vi "DPSK_RECV_TEST.vi"() -> ()   [LabVIEW 2020]
uses:
  <vilib>/Utility/error.llb/DialogType.ctl
  <instrlib>/niUSRP/niUSRP Fetch Rx Data (CDB WDT).vi
panel:
  in  "数据源文件":path=path "C:/Users/admin/Desktop/USRP0902/USRP/Dpsk/SendBit.mat"
  in  "接收码元速率":dbl=10000.0
  in  "信源比特长度":dbl=1000.0
  out "波形图":dbl[](graph)
  in  "Stop Button":bool
  in  "天线选择":string="RX2"
  out "实际接收增益":dbl=10.0 format="%#_6f"
  out "实际载波频率":dbl=1000000000.0 format="%#_6p"
  out "实际基带采样率":dbl=200000.0 format="%#_6p"
  in  "设定接收增益":dbl=10.0 format="%#_6f"
  in  "设定载波频率":dbl=1000000000.0 format="%#_6p"
  in  "设定基带采样率":dbl=200000.0 format="%#_6p"
  in  "设备IP":refnum<k15>="192.168.10.2"
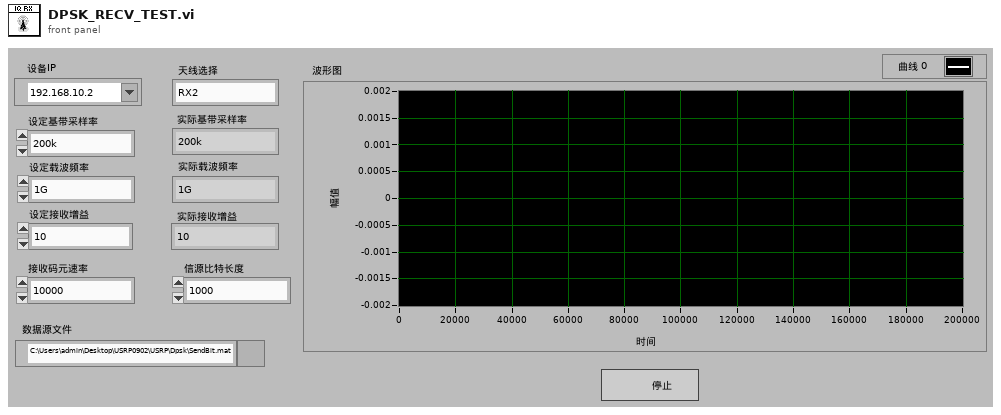
[diagram p1: front panel]
types:
  T1 = typedef "DialogType.ctl" = u16
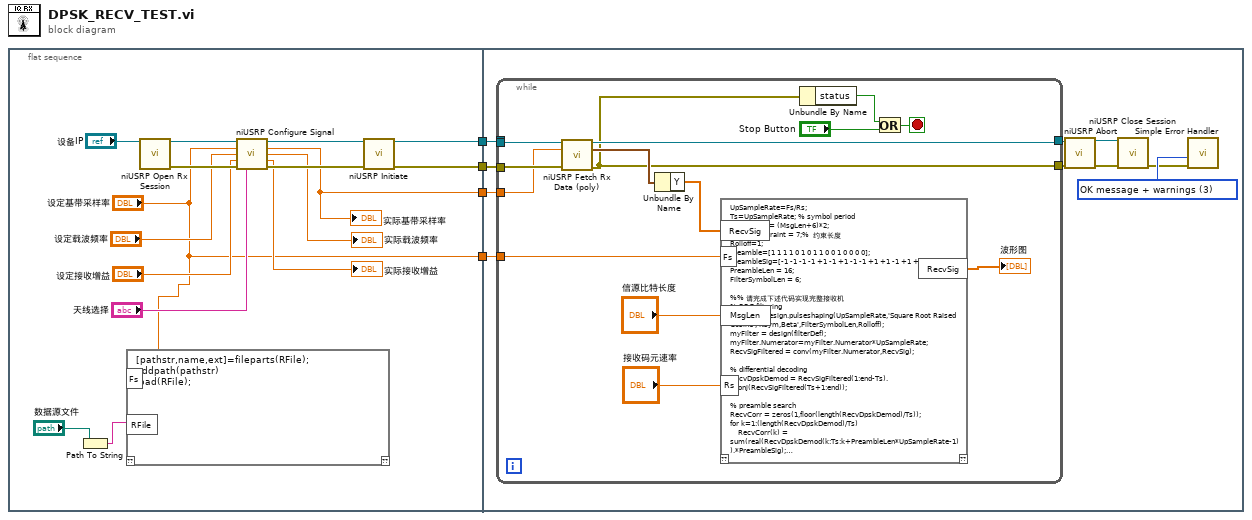
[diagram p0: block diagram]
diagram:
  n1 = flat-sequence {
    tunnel: [w11] -> w4
    tunnel: [w10] -> w3
    tunnel: ["设定基带采样率"] -> w2
    tunnel: [w9] -> w1
    tunnel: w4 -> [w26]
    tunnel: w3 -> [w25]
    tunnel: w2 -> [w22]
    tunnel: w1 -> [w21]
    frame #0 {
      n2 = Path To String(path="数据源文件") -> (string=w5:string)
      n3 = script code="[pathstr,name,ext]=fileparts(RFile);\naddpath(pathstr)\nload(RFile);"("Fs"="设定基带采样率", "RFile"=w5) -> ()  [unwired: 2 out]
      n4 = call <instrlib>:"niUSRP Open Rx Session.vi"("device names"="设备IP") -> ("session handle out"=w20:refnum<k15>, "error out"=w19:errorcluster)  [unwired: 13 in]
      n5 = call <instrlib>:"niUSRP Configure Signal.vi"("session handle"=w20, "IQ rate"="设定基带采样率", "carrier frequency"="设定载波频率", "gain"="设定接收增益", "error in (no error)"=w19, "active antenna"="天线选择") -> ("session handle out"=w14:refnum<k15>, "coerced IQ rate"=w9:dbl, "coerced carrier frequency"=→"实际载波频率":dbl, "coerced gain"=→"实际接收增益":dbl, "error out"=w16:errorcluster)  [unwired: 5 in]
      "实际基带采样率" <- w9
      n6 = call <instrlib>:"niUSRP Initiate.vi"("session handle"=w14, "error in (no error)"=w16) -> ("session handle out"=w11:refnum<k15>, "error out"=w10:errorcluster)  [unwired: 12 in]
    }
    frame #1 {
      w24 = T1 3 items=["no dialog", "OK message", "continue or stop message", "OK message + warnings", "continue/stop + warnings"] ("type of dialog (OK msg:1)")
      n7 = while {
        tunnel: [w38] -> _
        tunnel: [w43] -> w28
        tunnel: [w39] -> w27
        tunnel: w26 -> [w38]
        tunnel: w25 -> [w37]
        tunnel: w22 -> [w36]
        tunnel: w21 -> [w33]
        stop <- w42 stop-if-true
        n8 = call-poly <instrlib>:"niUSRP Fetch Rx Data (poly).vi"("session handle"=w38, "number of samples"=w33, "error in (no error)"=w37) -> ("session handle out"=w43:refnum<k15>, "data"=w40:waveform(cdb), "error out"=w39:errorcluster)  [unwired: 9 in, 1 out]
        n9 = Unbundle By Name ("Get Waveform Components")(w40) -> ("Y"=w35:cdb[])
        n10 = script code="UpSampleRate=Fs/Rs;\nTs=UpSampleRate; % symbol period\nSymbolLen = (MsgLen+6)*2;\nCoderConstraint = 7;%  约束长度 \nRolloff=1;\nPreamble=[1 1 1 1 0 1 0 1 1 0 0 1 0 0 0 0];\nPreambleSig=[-1 -1 -1 -1 +1 -1 +1 -1 -1 +1 +1 -1 +1 +1 +1 +1];\nPreambleLen = 16;\nFilterSymbolLen = 6;\n\n%% 请完成下述代码实现完整接收机\n% RRC filtering\nfilterDef=fdesign.pulseshaping(UpSampleRate,'Square Root Raised Cosine','Nsym,Beta',FilterSymbolLen,Rolloff);\nmyFilter = design(filterDef);\nmyFilter.Numerator=myFilter.Numerator*UpSampleRate;\nRecvSigFiltered = conv(myFilter.Numerator,RecvSig);\n\n% differential decoding\nRecvDpskDemod = RecvSigFiltered(1:end-Ts).*conj(RecvSigFiltered(Ts+1:end));  \n\n% preamble search\nRecvCorr = zeros(1,floor(length(RecvDpskDemod)/Ts));\nfor k=1:(length(RecvDpskDemod)/Ts)\n    RecvCorr(k) = sum(real(RecvDpskDemod(k:Ts:k+PreambleLen*UpSampleRate-1)).*PreambleSig);\nend\nRecvCorr = abs(RecvCorr);\n[~, pos ] = max(RecvCorr); \n\n% sampled symbol\nRecvSymbolSampled = RecvDpskDemod(pos:UpSampleRate:pos+(PreambleLen+SymbolLen)*UpSampleRate-1);    \nRecvSymbolSampled = real(sign(RecvSymbolSampled(PreambleLen+1:end)));\n\n% convolutoinal decoding\ntrel = poly2trellis(CoderConstraint, [171, 133]);\nRecvBit = vitdec(RecvSymbolSampled,trel,5*CoderConstraint,'term','unquant');\nRecvBit = RecvBit(1:length(RecvBit)-FilterSymbolLen);\n\nfigure(4);plot(real(RecvSig));title('real(RecvSig)：DPSK接收信号');\nfigure(5);plot(real(RecvSigFiltered));title('real(RecvSigFiltered)：滤波接收信号');\nfigure(6);plot(real(RecvDpskDemod));title('real(RecvDpskDemod)：DPSK解调后信号');\nfigure(7);plot(RecvCorr);title('RecvCorr：preamble相关结果');\nfigure(8);plot(real(RecvSymbolSampled));title('real(RecvSymbolSampled)：抽样码元');\nfigure(9);plot(RecvBit);title('RecvBit：译码比特');\nfigure(10);plot(abs(RecvBit-SendBit));title('abs(RecvBit-SendBit)：接收发送比特错误');"("RecvSig"=w35, "Fs"=w36, "MsgLen"="信源比特长度", "Rs"="接收码元速率") -> ("RecvSig"=→"波形图":cdb[])  [unwired: 2 out]
        n11 = Unbundle By Name(w39) -> ("status"=w44:bool)
        n12 = Or(x=w44, y="Stop Button") -> (x .or. y?=w42:bool)
      }
      n13 = call <instrlib>:"niUSRP Abort.vi"("session handle"=w28, "error in (no error)"=w27) -> ("session handle out"=w30:refnum<k15>, "error out"=w29:errorcluster)  [unwired: 12 in]
      n14 = call <instrlib>:"niUSRP Close Session.vi"("session handle"=w30, "error in (no error)"=w29) -> ("error out"=w23:errorcluster)  [unwired: 13 in]
      n15 = call <vilib>:"Simple Error Handler.vi"("type of dialog (OK msg:1)"=w24, "error in (no error)"=w23) -> ()  [unwired: 3 in, 5 out]
    }
  }
